vi "pack.vi"(8 "error in (no error)":errorcluster, 11 "Ao8FileReader in":refnum<class "Ao8FileReader.lvclass">) -> (0 "error out":errorcluster, 3 "Ao8FileReader out":refnum<class "Ao8FileReader.lvclass">)   [LabVIEW 2011, in "Tools.lvlib" / "Filing.lvlib" / "Ao8FileReader.lvclass"]
uses:
  Ao8FileReader.lvclass
  Ao8FileReader.lvclass/Ao8FileReader.ctl
  FileReader.lvclass
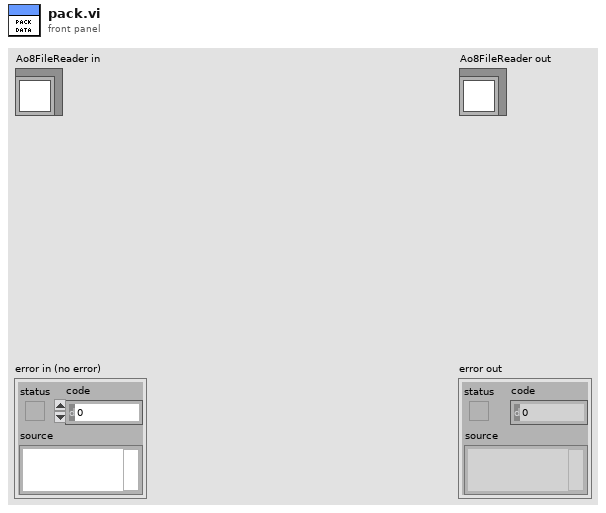
[diagram p1: front panel]
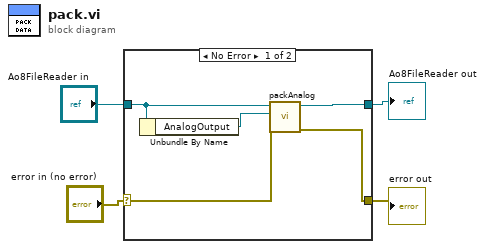
[diagram p0: block diagram]
diagram:
  n1 = case shown="No Error" "error in (no error)" {
    selector: "error in (no error)" -> [w8 w10]
    tunnel: [w9 w11] -> w4
    tunnel: "Ao8FileReader in" -> [w6 w11]
    tunnel: [w7 w10] -> w1
    frame No Error {
      n2 = Unbundle By Name(w6) -> ("AnalogOutput"=w5:refnum<class "AnalogOutput.lvclass">)
      n3 = call "packAnalog.vi"("error in (no error)"=w8, "AnalogOutput"=w5, "FileReader in"=w6) -> ("error out"=w7:errorcluster, "FileReader out"=w9:refnum<class "Ao8FileReader.lvclass">)  [unwired: 7 in]
    }
    frame Error {
    }
  }
  "error out" <- w1
  "Ao8FileReader out" <- w4
